vi "SWERVE_DRIVE_MODULE_ACT.vi"(6 "Pass_Through_Time":dbl=-1.0 format="%33.4f", 8 "SwervePosInDeadband":bool=TRUE, 9 "Swerve State":T1={"Speed"=0.0, "Angle"={"VALUE"=0.0, "COS"=1.0, "SIN"=0.0}} {"Angle"."SIN" format="%13.4f"; "Angle"."COS" format="%13.4f"; "Angle"."VALUE" format="%13.4f"}, 10 "Swerve Dmd":T1={"Speed"=0.0, "Angle"={"VALUE"=0.0, "COS"=1.0, "SIN"=0.0}} {"Angle"."SIN" format="%13.4f"; "Angle"."COS" format="%13.4f"; "Angle"."VALUE" format="%13.4f"}, 11 "Swerve Module TypDef":T3) -> (0 "SwerveOnTarget":bool, 1 "SwervePosError":dbl, 2 "Swerve Motor Dmd":dbl, 3 "Wheel Motor Dmd":dbl, 4 "WheelSpeedErr":dbl)   [LabVIEW 2019]
uses:
  SWERVE_DRIVE_MODULE_TYPDEF.ctl
  <vilib>/Rock Robotics/WPI/MotorControl/WPI_MotorControlDeviceRef.ctl
  <vilib>/Rock Robotics/WPI/MotorControl/WPI_MotorControlType.ctl
  <vilib>/Rock Robotics/SystemInterfaces/DIO/FPGA_DIOPWMChannel.ctl
  <vilib>/Rock Robotics/WPI/PWM/WPI_PWMDeadband.ctl
  <vilib>/Rock Robotics/SystemInterfaces/DIO/FPGA_DIOChannel.ctl
  <vilib>/Rock Robotics/WPI/Encoder/WPI_EncoderDevRef.ctl
  <vilib>/Rock Robotics/SystemInterfaces/Encoder/FPGA_EncoderIdx.ctl
  <vilib>/Rock Robotics/SystemInterfaces/Counter/FPGA_CounterCtrSystemIndex.ctl
  <vilib>/Rock Robotics/WPI/Encoder/WPI_EncoderType.ctl
  <vilib>/Rock Robotics/WPI/ThirdParty/JAS_Junk/TrajLib/TypeDef/SWERVE_DRIVE_MODULE_STATE.ctl
  <vilib>/Rock Robotics/WPI/ThirdParty/JAS_Junk/TrajLib/TypeDef/ROTATION2D.ctl
  <vilib>/Rock Robotics/WPI/ThirdParty/JAS_Junk/TrajLib/TypeDef/X_Y_PAIR.ctl
  <vilib>/Rock Robotics/WPI/ThirdParty/JAS_Junk/TrajLib/VI/Util_GetTime_U32.vi
  <vilib>/Rock Robotics/WPI/ThirdParty/JAS_Junk/TrajLib/MathUtil_InputModulus.vi
  <vilib>/Rock Robotics/WPI/ThirdParty/JAS_Junk/TrajLib/Rotation2d_Minus.vi
  <vilib>/Rock Robotics/WPI/ThirdParty/JAS_Junk/TrajLib/Rotation2d_GetRadians.vi
  <vilib>/Rock Robotics/WPI/ThirdParty/JAS_Junk/TrajLib/SwerveModuleState_New.vi
  <vilib>/Rock Robotics/WPI/ThirdParty/JAS_Junk/TrajLib/Rotation2d_RotateBy.vi
  <vilib>/Rock Robotics/WPI/ThirdParty/JAS_Junk/TrajLib/Rotation2d_CreateAngle.vi
  <vilib>/Rock Robotics/WPI/ThirdParty/JAS_Junk/TrajLib/ProfiledPIDController_SetPID.vi
  <vilib>/Rock Robotics/WPI/ThirdParty/JAS_Junk/TrajLib/ProfiledPIDController_SetIntegratorRange.vi
  <vilib>/Rock Robotics/WPI/ThirdParty/JAS_Junk/TrajLib/ProfiledPIDController_SetTolerance_PosVel.vi
  <vilib>/Rock Robotics/WPI/ThirdParty/JAS_Junk/TrajLib/ProfiledPIDController_DisableContInput.vi
  <vilib>/Rock Robotics/WPI/ThirdParty/JAS_Junk/TrajLib/ProfiledPIDController_EnableContInput.vi
  <vilib>/Rock Robotics/WPI/ThirdParty/JAS_Junk/TrajLib/ProfiledPIDController_Reset_PosOnly.vi
  <vilib>/Rock Robotics/WPI/ThirdParty/JAS_Junk/TrajLib/ProfiledPIDController_NewPeriod.vi
  <vilib>/Rock Robotics/WPI/ThirdParty/JAS_Junk/TrajLib/ProfiledPIDController_Calculate_Meas_Goal.vi
  <vilib>/Rock Robotics/WPI/ThirdParty/JAS_Junk/TrajLib/ProfiledPIDController_AtGoal.vi
  <vilib>/Rock Robotics/WPI/ThirdParty/JAS_Junk/TrajLib/ProfiledPIDController_AtSetpoint.vi
  <vilib>/Rock Robotics/WPI/ThirdParty/JAS_Junk/TrajLib/ProfiledPIDController_SetConstraints.vi
  <vilib>/Rock Robotics/WPI/ThirdParty/JAS_Junk/TrajLib/VI/FunctionGenerator_New.vi
  <vilib>/Rock Robotics/WPI/ThirdParty/JAS_Junk/TrajLib/VI/FunctionGenerator_Calculate.vi
  <vilib>/Rock Robotics/WPI/ThirdParty/JAS_Junk/TrajLib/PIDController_AtSetpoint.vi
  <vilib>/Rock Robotics/WPI/ThirdParty/JAS_Junk/TrajLib/PIDController_SetPIDF.vi
  <vilib>/Rock Robotics/WPI/ThirdParty/JAS_Junk/TrajLib/PIDController_SetDerivativeFilter.vi
  <vilib>/Rock Robotics/WPI/ThirdParty/JAS_Junk/TrajLib/PIDController_SetIntegratorRange.vi
  <vilib>/Rock Robotics/WPI/ThirdParty/JAS_Junk/TrajLib/PIDController_SetTolerancePandV.vi
  <vilib>/Rock Robotics/WPI/ThirdParty/JAS_Junk/TrajLib/PIDController_DisableContinousInput.vi
  <vilib>/Rock Robotics/WPI/ThirdParty/JAS_Junk/TrajLib/PIDController_EnableContinousInput.vi
  <vilib>/Rock Robotics/WPI/ThirdParty/JAS_Junk/TrajLib/PIDController_Reset.vi
  <vilib>/Rock Robotics/WPI/ThirdParty/JAS_Junk/TrajLib/PIDController_New.vi
  <vilib>/Rock Robotics/WPI/ThirdParty/JAS_Junk/TrajLib/PIDController_SetOutputLimits.vi
  <vilib>/Rock Robotics/WPI/ThirdParty/JAS_Junk/TrajLib/SlewRateLimiter_New.vi
  <vilib>/Rock Robotics/WPI/ThirdParty/JAS_Junk/TrajLib/SlewRateLimiter_Reset.vi
  <vilib>/Rock Robotics/WPI/ThirdParty/JAS_Junk/TrajLib/SlewRateLimiter_Calculate.vi
  <vilib>/Rock Robotics/WPI/ThirdParty/JAS_Junk/TrajLib/SlewRateLimiter_SetRate.vi
  <vilib>/Rock Robotics/WPI/ThirdParty/JAS_Junk/TrajLib/Rotation2d_UnaryMinus.vi
  <vilib>/Rock Robotics/WPI/ThirdParty/JAS_Junk/TrajLib/Rotation2d_CreateXY.vi
  <vilib>/Rock Robotics/WPI/ThirdParty/JAS_Junk/TrajLib/PIDController_SetPID.vi
  <vilib>/Rock Robotics/WPI/ThirdParty/JAS_Junk/TrajLib/TrapProfState_New.vi
  <vilib>/Rock Robotics/WPI/ThirdParty/JAS_Junk/TrajLib/ProfiledPIDController_Reset.vi
  <vilib>/Rock Robotics/WPI/ThirdParty/JAS_Junk/TrajLib/PIDController_NewPeriod.vi
  <vilib>/Rock Robotics/SystemInterfaces/NetworkCommunication/NetComm_UsageReport_report.vi
  <vilib>/Rock Robotics/WPI/ThirdParty/JAS_Junk/TrajLib/ProfiledPIDController_SetGoal_PosOnly.vi
  <vilib>/Rock Robotics/WPI/ThirdParty/JAS_Junk/TrajLib/ProfiledPIDController_Calculate_Meas.vi
  <vilib>/Rock Robotics/WPI/ThirdParty/JAS_Junk/TrajLib/TrapProfState_Equals.vi
  <vilib>/Rock Robotics/WPI/ThirdParty/JAS_Junk/TrajLib/Util_CalcDist.vi
  <vilib>/Rock Robotics/WPI/ThirdParty/JAS_Junk/TrajLib/ProfiledPIDController_SetGoal.vi
  <vilib>/Rock Robotics/WPI/ThirdParty/JAS_Junk/TrajLib/PIDController_Calculate_SP_PV.vi
  <vilib>/Rock Robotics/WPI/ThirdParty/JAS_Junk/TrajLib/TrapProfile_New.vi
  <vilib>/Rock Robotics/WPI/ThirdParty/JAS_Junk/TrajLib/ProfiledPIDController_GetPeriod.vi
  <vilib>/Rock Robotics/WPI/ThirdParty/JAS_Junk/TrajLib/TrapProfile_Calculate.vi
  <vilib>/Rock Robotics/WPI/ThirdParty/JAS_Junk/TrajLib/ControllerUtil_GetModulusError.vi
  <vilib>/Rock Robotics/WPI/ThirdParty/JAS_Junk/TrajLib/PIDController_SetSetpoint.vi
  <vilib>/Rock Robotics/WPI/ThirdParty/JAS_Junk/TrajLib/PIDController_Calculate_PV.vi
  <vilib>/Rock Robotics/WPI/ThirdParty/JAS_Junk/TrajLib/TrapProfile_ShouldFlipAcceleration.vi
  <vilib>/Rock Robotics/WPI/ThirdParty/JAS_Junk/TrajLib/TrapProfile_Direct.vi
  <vilib>/Rock Robotics/WPI/ThirdParty/JAS_Junk/TrajLib/PIDController_GetPeriod.vi
  <vilib>/gmath/interp.llb/Search Ordered Table.vi
  <vilib>/Rock Robotics/WPI/ThirdParty/JAS_Junk/TrajLib/VI/Util_GetTime_U64.vi
  <vilib>/Rock Robotics/WPI/ThirdParty/JAS_Junk/TrajLib/Globals/Util_LibraryGlobals.vi
  <vilib>/Rock Robotics/WPI/ThirdParty/JAS_Junk/TrajLib/PIDController_AdvCalculate_FF_Sp_Pv.vi
  <vilib>/Rock Robotics/WPI/ThirdParty/JAS_Junk/TrajLib/Trajectory_Library.lvlib
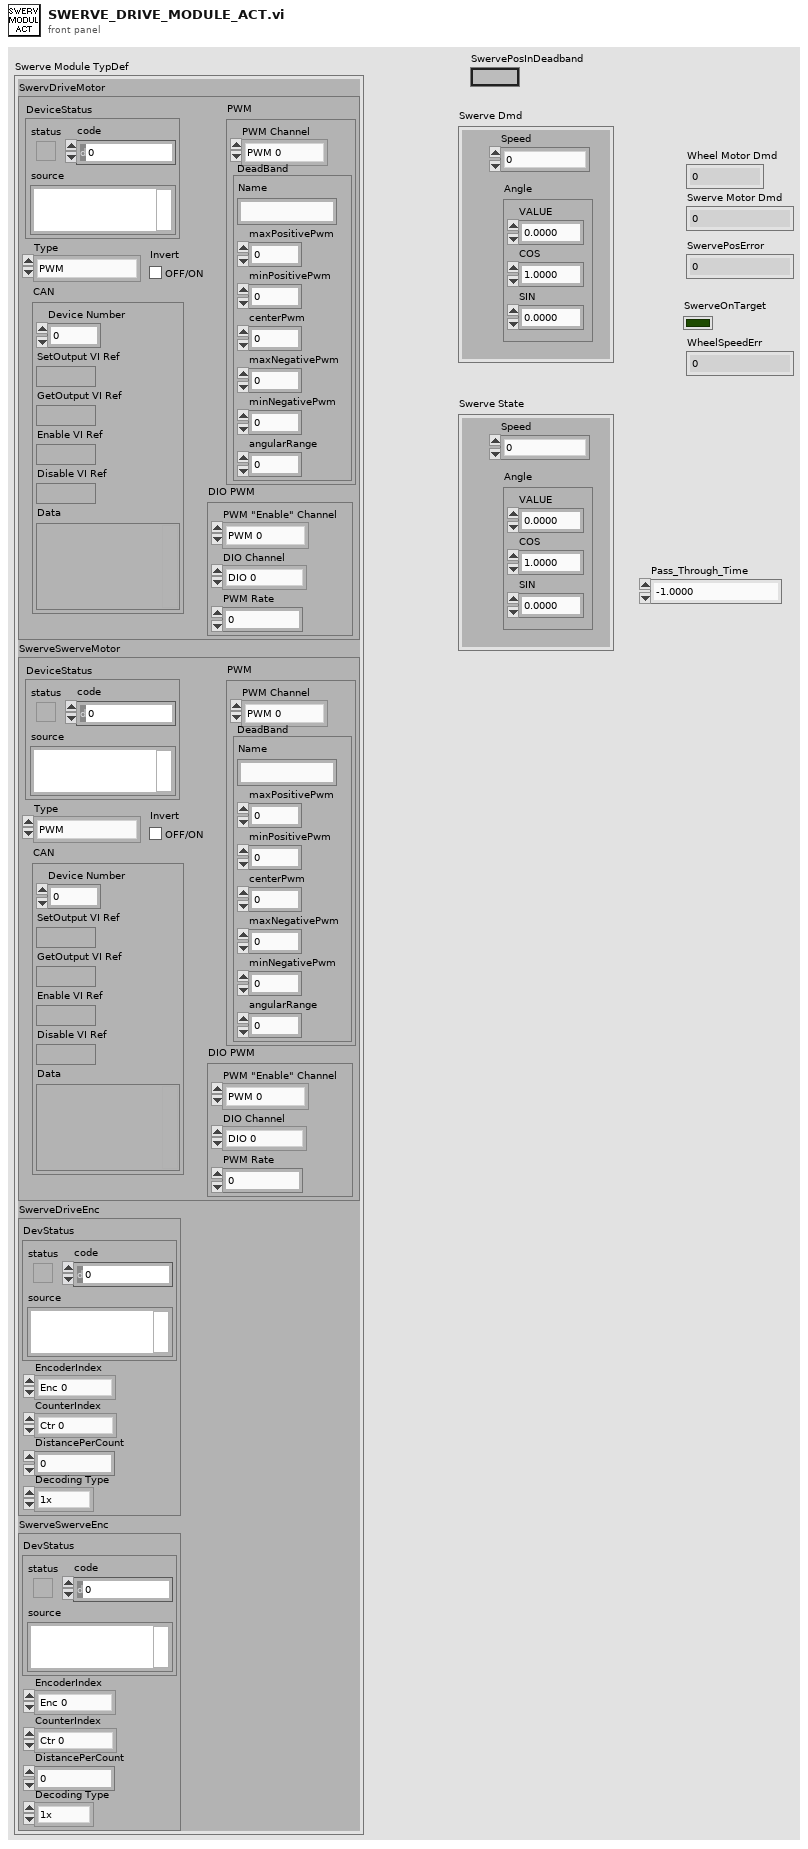
[diagram p1: front panel]
types:
  T1 = typedef "Trajectory_Library.lvlib/SWERVE_DRIVE_MODULE_STATE.ctl" = cluster{"Speed":dbl, "Angle":T2}
  T2 = typedef "Trajectory_Library.lvlib/ROTATION2D.ctl" = cluster{"VALUE":dbl, "COS":dbl, "SIN":dbl}
  T3 = typedef "SWERVE_DRIVE_MODULE_TYPDEF.ctl" = cluster{"SwervDriveMotor":T4, "SwerveSwerveMotor":T4, "SwerveDriveEnc":T9, "SwerveSwerveEnc":T9}
  T4 = typedef "WPI_MotorControlDeviceRef.ctl" = cluster{"DeviceStatus":errorcluster, "Type":T5, "PWM":cluster{"PWM Channel":T6, "DeadBand":T7}, "CAN":cluster{"Device Number":u8, "SetOutput VI Ref":variant, "GetOutput VI Ref":variant, "Enable VI Ref":variant, "Disable VI Ref":variant, "Data":variant}, "Invert":bool, "DIO PWM":cluster{"PWM \"Enable\" Channel":T6, "DIOChannel":T8, "PWM Rate":dbl}}
  T5 = typedef "WPI_MotorControlType.ctl" = enum16{"PWM", "CAN", "DIO PWM"}
  T6 = typedef "FPGA_DIOPWMChannel.ctl" = enum8{"PWM 0", "PWM 1", "PWM 2", "PWM 3", "PWM 4", "PWM 5", "PWM 6", "PWM 7", "PWM 8", "PWM 9", "PWM MXP 0", "PWM MXP 1", "PWM MXP 2", "PWM MXP 3", "PWM MXP 4", "PWM MXP 5", "PWM MXP 6", "PWM MXP 7", "PWM MXP 8", "PWM MXP 9", "Invalid"}
  T7 = typedef "WPI_PWMDeadband.ctl" = cluster{"Name":string, "maxPositivePwm":i32, "minPositivePwm":i32, "centerPwm":i32, "maxNegativePwm":i32, "minNegativePwm":i32, "angularRange":u16}
  T8 = typedef "FPGA_DIOChannel.ctl" = enum8{"DIO 0", "DIO 1", "DIO 2", "DIO 3", "DIO 4", "DIO 5", "DIO 6", "DIO 7", "DIO 8", "DIO 9", "DIO MXP 0", "DIO MXP 1", "DIO MXP 2", "DIO MXP 3", "DIO MXP 4", "DIO MXP 5", "DIO MXP 6", "DIO MXP 7", "DIO MXP 8", "DIO MXP 9", "DIO MXP 10", "DIO MXP 11", "DIO MXP 12", "DIO MXP 13", "DIO MXP 14", "DIO MXP 15", "SPI Port CS1", "SPI Port CS2", "SPI Port CS3", "SPI Port MISO", "SPI Port MOSI", "Invalid"}
  T9 = typedef "WPI_EncoderDevRef.ctl" = cluster{"DevStatus":errorcluster, "EncoderIndex":T10, "CounterIndex":T11, "DistancePerCount":dbl, "Decoding Type":T12}
  T10 = typedef "FPGA_EncoderIdx.ctl" = enum8{"Enc 0", "Enc 1", "Enc 2", "Enc 3", "Enc 4", "Enc 5", "Enc 6", "Enc 7", "Invalid"}
  T11 = typedef "FPGA_CounterCtrSystemIndex.ctl" = enum8{"Ctr 0", "Ctr 1", "Ctr 2", "Ctr 3", "Ctr 4", "Ctr 5", "Ctr 6", "Ctr 7", "Invalid"}
  T12 = typedef "WPI_EncoderType.ctl" = enum16{"1x", "2x", "4x"}
  T13 = typedef "Trajectory_Library.lvlib/X_Y_PAIR.ctl" = cluster{"X":dbl, "Y":dbl}
  T14 = typedef "Trajectory_Library.lvlib/PID_ADV_LIMITS.ctl" = cluster{"MaxInput":dbl, "MinInput":dbl, "Continuous":bool, "MaxOutput":dbl, "MinOutput":dbl}
  T15 = typedef "Trajectory_Library.lvlib/PID_ADV_TUNING.ctl" = cluster{"Kf":dbl, "Kp":dbl, "Ki":dbl, "Kd":dbl, "MaximumIntegral":dbl, "MinimumIntegral":dbl, "Filter Derivative":bool}
  T16 = typedef "Trajectory_Library.lvlib/PID_CONTROLLER.ctl" = cluster{"Kp":dbl, "Ki":dbl, "Kd":dbl, "Period":dbl, "Max_Integral":dbl, "Min_Integral":dbl, "Max_Input":dbl, "Min_Input":dbl, "Continuous":bool, "PositionError":dbl, "VelocityError":dbl, "PrevError":dbl, "TotalError":dbl, "PositionTolerance":dbl, "VelocityTolerance":dbl, "SetPoint":dbl, "Kf":dbl, "Prev_Deriv":dbl, "Prev_Deriv 2":dbl, "DerivativeFilter":bool, "Min_Output":dbl, "Max_Output":dbl, "Prev_F_P":dbl, "Prev_F_P_2":dbl, "AntiWindupActive":bool, "Measurement":dbl}
  T17 = typedef "Trajectory_Library.lvlib/PID_TUNING.ctl" = cluster{"Kp":dbl, "Ki":dbl, "Kd":dbl, "MaximumIntegral":dbl, "MinimumIntegral":dbl}
  T18 = typedef "Trajectory_Library.lvlib/PID_ERROR_TOLERANCE.ctl" = cluster{"PositionTolerance":dbl, "VelocityTolerance":dbl}
  T19 = typedef "Trajectory_Library.lvlib/PID_INPUT_LIMITS.ctl" = cluster{"MaxInput":dbl, "MinInput":dbl, "Continuous":bool}
  T20 = typedef "Trajectory_Library.lvlib/TRAPEZOID_PROFILE_CONSTRAINT.ctl" = cluster{"MaxVelocity":dbl, "MaxAcceleration":dbl}
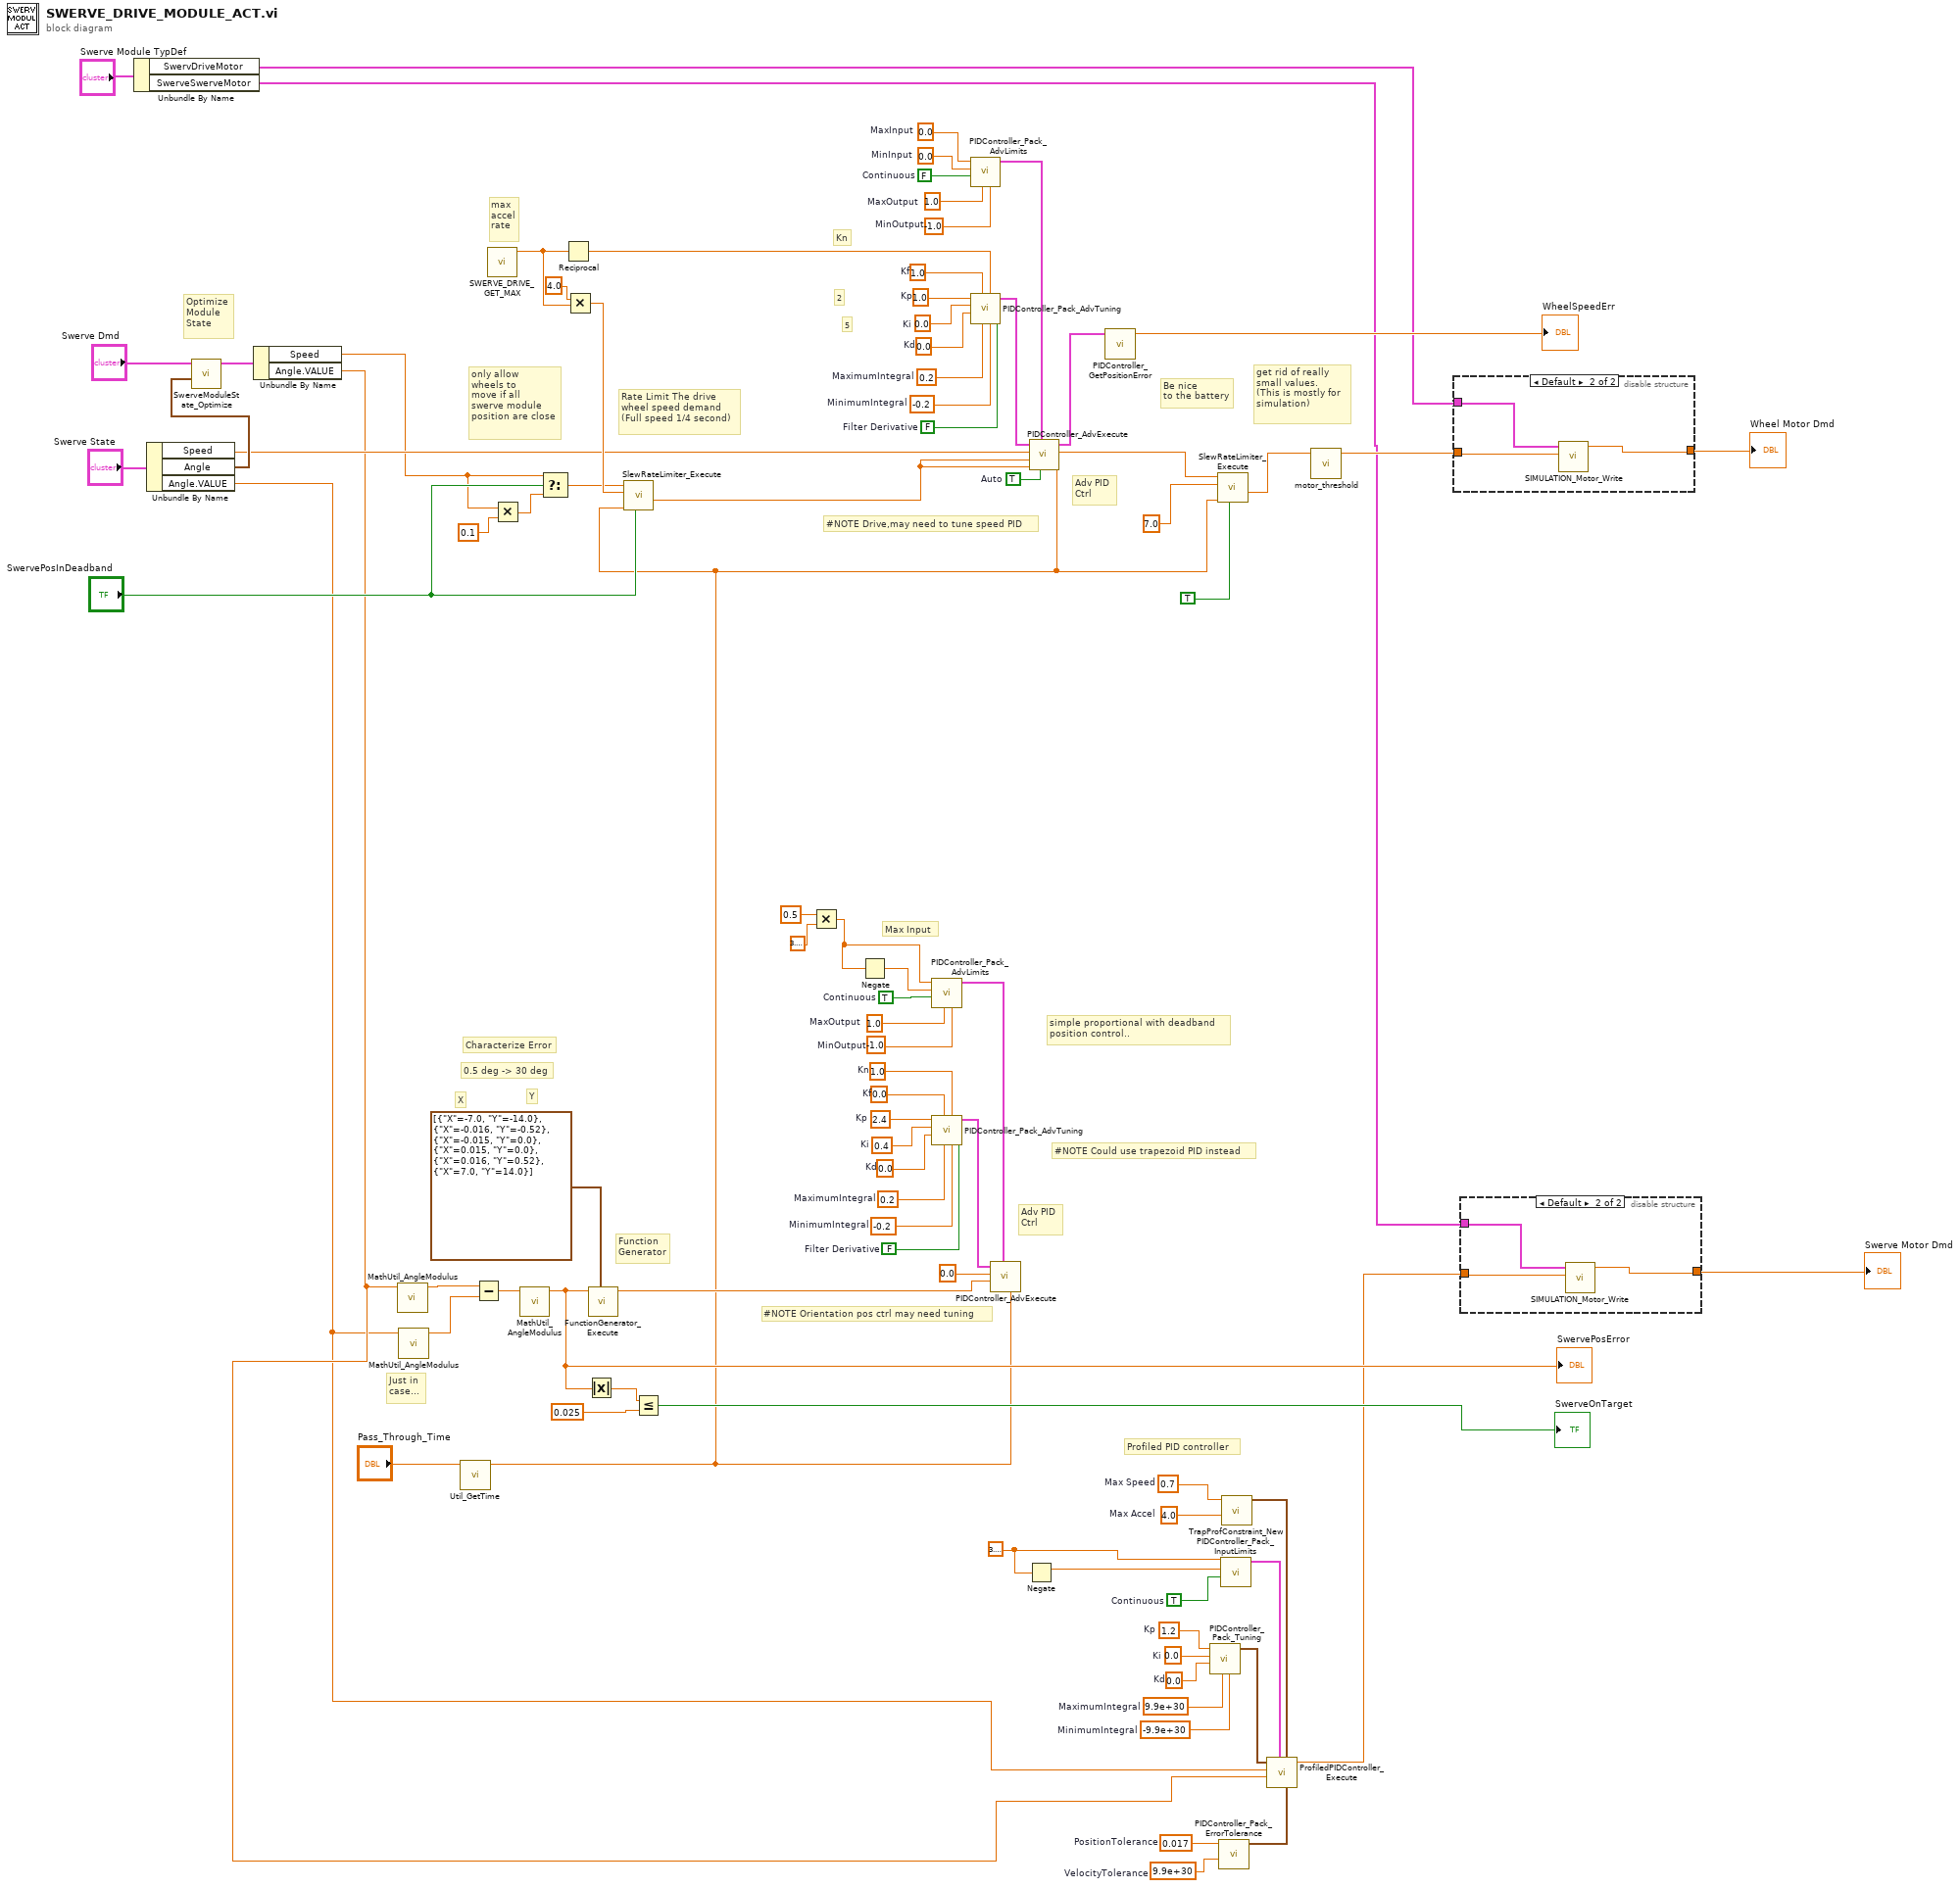
[diagram p0: block diagram]
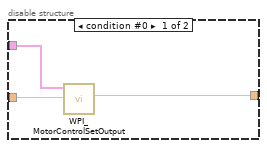
[diagram p2: hidden frame]
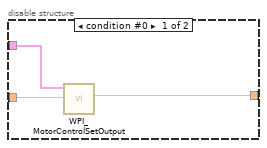
[diagram p3: hidden frame]
diagram:
  w15 = 3.141592653589793
  w30 = 0.017  # PositionTolerance
  w29 = 9.9e+30  # VelocityTolerance
  w27 = 0.7  # Max Speed
  w26 = 4.0  # Max Accel
  w24 = TRUE  # Continuous
  w23 = 1.2  # Kp
  w22 = 0.0  # Ki
  w21 = 0.0  # Kd
  w20 = 9.9e+30  # MaximumIntegral
  w19 = -9.9e+30  # MinimumIntegral
  w39 = TRUE  # Auto
  w55 = 1.0  # Kp
  w54 = 0.0  # Ki
  w53 = 0.0  # Kd
  w52 = 1.0  # Kf
  w51 = 0.2  # MaximumIntegral
  w50 = -0.2  # MinimumIntegral
  w49 = FALSE  # Filter Derivative
  w47 = 0.0  # MinInput
  w46 = FALSE  # Continuous
  w45 = 1.0  # MaxOutput
  w48 = -1.0  # MinOutput
  w44 = 0.0  # MaxInput
  w68 = 1.0  # MaxOutput
  w69 = -1.0  # MinOutput
  w83 = 1.0  # Kn
  w82 = 2.4  # Kp
  w81 = 0.4  # Ki
  w80 = 0.0  # Kd
  w79 = 0.0  # Kf
  w78 = 0.2  # MaximumIntegral
  w77 = -0.2  # MinimumIntegral
  w76 = FALSE  # Filter Derivative
  w75 = TRUE  # Continuous
  # "Be nice\nto the battery"
  # "5"
  # "2"
  # "Profiled PID controller"
  # "Optimize\nModule\nState"
  # "Kn"
  # "Adv PID\nCtrl"
  # "Rate Limit The drive\nwheel speed demand\n(Full speed 1/4 second)"
  # "Just in \ncase..."
  # "#NOTE Could use trapezoid PID instead"
  # "Characterize Error"
  # "Max Input"
  # "Adv PID\nCtrl"
  # "0.5 deg -> 30 deg"
  # "Function\nGenerator"
  # "Y"
  # "X"
  # "#NOTE Orientation pos ctrl may need tuning"
  # "only allow\nwheels to \nmove if all \nswerve module \nposition are close"
  # "#NOTE Drive,may need to tune speed PID"
  # "simple proportional with deadband\nposition control.."
  # "get rid of really\nsmall values.\n(This is mostly for \nsimulation)"
  # "max\naccel\nrate"
  n1 = Unbundle By Name("Swerve Module TypDef") -> ("SwervDriveMotor"=w35:T4, "SwerveSwerveMotor"=w33:T4)
  n2 = Unbundle By Name("Swerve State") -> ("Speed"=w40:dbl, "Angle"=w58:T2, "Angle.VALUE"=w13:dbl)
  n3 = call <vilib>:"SwerveModuleState_Optimize.vi"("CurrentAngle"=w58, "Desired State"="Swerve Dmd") -> ("out SWERVE_DRIVE_MODULE_STATE"=w57:T1)  [unwired: 9 in]
  n4 = Unbundle By Name(w57) -> ("Speed"=w6:dbl, "Angle.VALUE"=w14:dbl)
  n5 = call <vilib>:"MathUtil_AngleModulus.vi"("InputAngle"=w14) -> ("ModulsAngle"=w63:dbl)  [unwired: 10 in]
  n6 = call <vilib>:"MathUtil_AngleModulus.vi"("InputAngle"=w13) -> ("ModulsAngle"=w62:dbl)  [unwired: 10 in]
  n7 = call <vilib>:"Util_GetTime.vi"("Pass_Through_Time"="Pass_Through_Time") -> ("FPGA_Time_Seconds"=w8:dbl)  [unwired: 8 in, 2 out]
  n8 = Subtract(x=w63, y=w62) -> (x-y=w64:dbl)
  n9 = call "SWERVE_DRIVE_GET_MAX.vi"() -> ("Max Wheel Vel (Meter/Sec)"=w88:dbl)  [unwired: 10 in, 1 out]
  n10 = Multiply(x=w6, y=0.1) -> (x*y=w4:dbl)
  n11 = call <vilib>:"MathUtil_AngleModulus.vi"("InputAngle"=w64) -> ("ModulsAngle"=w61:dbl)  [unwired: 10 in]
  "SwervePosError" <- w61
  n12 = Select(t=w6, s="SwervePosInDeadband", f=w4) -> (s? t:f=w85:dbl)
  n13 = Reciprocal(x=w88) -> (1/x=w41:dbl)
  n14 = Multiply(x=4.0, y=w88) -> (x*y=w86:dbl)
  n15 = Absolute Value(x=w61) -> (abs(x)=w67:dbl)
  n16 = call <vilib>:"FunctionGenerator_Execute.vi"("X Y Pairs"=T13[] [{"X"=-7.0, "Y"=-14.0}, {"X"=-0.016, "Y"=-0.52}, {"X"=-0.015, "Y"=0.0}, {"X"=0.015, "Y"=0.0}, {"X"=0.016, "Y"=0.52}, {"X"=7.0, "Y"=14.0}], "Input Value"=w61) -> ("Output Value"=w70:dbl)  [unwired: 9 in]
  n17 = call <vilib>:"SlewRateLimiter_Execute.vi"("Enable"="SwervePosInDeadband", "Time"=w8, "PositiveRate"=w86, "Input"=w85) -> ("Output"=w36:dbl)  [unwired: 6 in, 1 out]
  n18 = Less Or Equal?(x=w67, y=0.025 ("ErrDeadband")) -> (x <= y?=→"SwerveOnTarget":bool)
  n19 = Multiply(x=0.5, y=3.141592653589793) -> (x*y=w3:dbl)
  n20 = Negate(x=w3) -> (-x=w72:dbl)
  n21 = call <vilib>:"PIDController_Pack_AdvLimits.vi"("MinOutput"=w69, "MaxOutput"=w68, "Continuous"=w75, "MinInput"=w72, "MaxInput"=w3) -> ("Adv PID Limits"=w73:T14)  [unwired: 6 in]
  n22 = call <vilib>:"PIDController_Pack_AdvTuning.vi"("Filter Derivative"=w76, "MinimumIntegral"=w77, "Kn"=w83, "MaximumIntegral"=w78, "Kf"=w79, "Kd"=w80, "Ki"=w81, "Kp"=w82) -> ("Adv PID Tuning"=w74:T15)  [unwired: 3 in]
  n23 = call <vilib>:"PIDController_Pack_AdvLimits.vi"("MinOutput"=w48, "MaxOutput"=w45, "Continuous"=w46, "MinInput"=w47, "MaxInput"=w44) -> ("Adv PID Limits"=w42:T14)  [unwired: 6 in]
  n24 = call <vilib>:"PIDController_Pack_AdvTuning.vi"("Filter Derivative"=w49, "MinimumIntegral"=w50, "Kn"=w41, "MaximumIntegral"=w51, "Kf"=w52, "Kd"=w53, "Ki"=w54, "Kp"=w55) -> ("Adv PID Tuning"=w43:T15)  [unwired: 3 in]
  n25 = call <vilib>:"PIDController_AdvExecute.vi"("Time"=w8, "Adv PID Limits"=w73, "SP-SetPoint"=w70, "PV-Measurement"=0.0, "Adv PID Tuning"=w74) -> ()  [unwired: 4 in, 3 out]
  n26 = Negate(x=w15) -> (-x=w16:dbl)
  n27 = call <vilib>:"PIDController_AdvExecute.vi"("Time"=w8, "Auto"=w39, "Adv PID Limits"=w42, "FF-FeedForward"=w36, "SP-SetPoint"=w36, "PV-Measurement"=w40, "Adv PID Tuning"=w43) -> ("CO-ControlOutput"=w11:dbl, "out PID_CONTROLLER"=w38:T16)  [unwired: 2 in, 1 out]
  n28 = call <vilib>:"PIDController_GetPositionError.vi"("in PID_CONTROLLER"=w38) -> ("PositionError"=→"WheelSpeedErr":dbl)  [unwired: 10 in]
  n29 = call <vilib>:"PIDController_Pack_Tuning.vi"("MinimumIntegral"=w19, "MaximumIntegral"=w20, "Kd"=w21, "Ki"=w22, "Kp"=w23) -> ("PID Tuning"=w18:T17)  [unwired: 6 in]
  n30 = call <vilib>:"SlewRateLimiter_Execute.vi"("Enable"=TRUE, "Time"=w8, "PositiveRate"=7.0, "Input"=w11) -> ("Output"=w10:dbl)  [unwired: 6 in, 1 out]
  n31 = call <vilib>:"PIDController_Pack_ErrorTolerance.vi"("VelocityTolerance"=w29, "PositionTolerance"=w30) -> ("PID Error Tolerance"=w28:T18)  [unwired: 9 in]
  n32 = call <vilib>:"PIDController_Pack_InputLimits.vi"("Continuous"=w24, "MinInput"=w16, "MaxInput"=w15) -> ("PID Input Limits"=w17:T19)  [unwired: 8 in]
  n33 = call <vilib>:"TrapProfConstraint_New.vi"("Max Accel"=w26, "Max Speed (M/S)"=w27) -> ("TRAPEZOID_PROFILE_CONSTRAINT"=w25:T20)  [unwired: 9 in]
  n34 = call <vilib>:"ProfiledPIDController_Execute.vi"("PID Error Tolerance"=w28, "Constraints"=w25, "PID Input Limits"=w17, "SP-SetPoint Goal"=w14, "PV-Measurement"=w13, "PID Tuning"=w18) -> ("CO-ControlOutput"=w12:dbl)  [unwired: 2 in, 3 out]
  n35 = call "motor_threshold.vi"("motor in"=w10) -> ("motor out"=w34:dbl)  [unwired: 10 in]
  n36 = disable-structure shown="Default" {
    disable-tunnel: w34 -> [w93 w95]
    disable-tunnel: w35 -> [w92 w96]
    disable-tunnel: [w91 w94] -> w32
    frame condition #0 {
      n37 = call <vilib>:"WPI_MotorControlSetOutput.vi"("Output"=w93, "MotorControlDevRef"=w92) -> ("Motor Output"=w91:dbl)  [unwired: 7 in, 2 out]
    }
    frame condition #1 (active) {
      n38 = call "SIMULATION_Motor_Write.vi"("Motor Demand"=w95, "Motor Device Reference"=w96) -> ("Out Motor Demand"=w94:dbl)  [unwired: 9 in]
    }
  }
  "Wheel Motor Dmd" <- w32
  n39 = disable-structure shown="Default" {
    disable-tunnel: w12 -> [w99 w101]
    disable-tunnel: w33 -> [w98 w102]
    disable-tunnel: [w97 w100] -> w31
    frame condition #0 {
      n40 = call <vilib>:"WPI_MotorControlSetOutput.vi"("Output"=w99, "MotorControlDevRef"=w98) -> ("Motor Output"=w97:dbl)  [unwired: 7 in, 2 out]
    }
    frame condition #1 (active) {
      n41 = call "SIMULATION_Motor_Write.vi"("Motor Demand"=w101, "Motor Device Reference"=w102) -> ("Out Motor Demand"=w100:dbl)  [unwired: 9 in]
    }
  }
  "Swerve Motor Dmd" <- w31
